vi "Calculate ANN.vi"(1 "1D ANN":i32[](array[numeric]), 2 "3D W":sgl[][][](array[numeric]) format="%.2f", 3 "Inputs":sgl[](array[numeric]) format="%.2f", 4 "Function":enum16{"Linear", "Sigmoid", "Tangent hyp."}(ring)) -> (7 "Neurons ouputs":sgl[][](array[numeric]) format="%.2f")   [LabVIEW 2010]
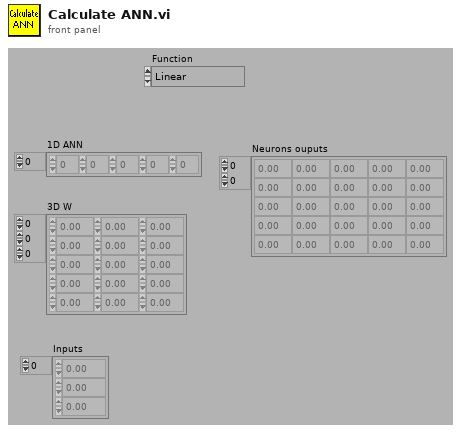
[diagram p1: front panel]
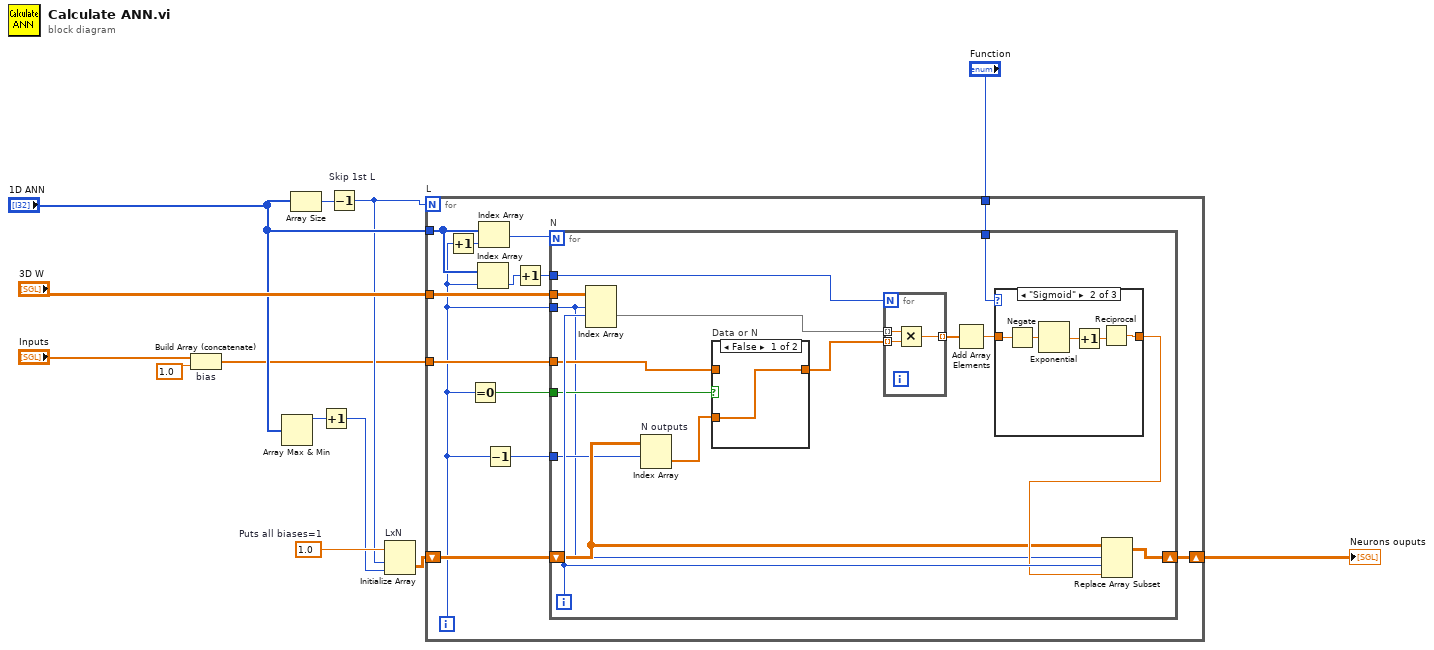
[diagram p0: block diagram]
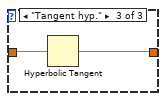
[diagram p3: hidden frame]
diagram:
  w7 = sgl 1.0  # Puts all biases=1
  n1 = Build Array (concatenate) "bias"("Inputs", sgl 1.0 ("Input Element")) -> (w1:sgl[])
  n2 = Array Max & Min(array="1D ANN") -> (max value=w5:i32)  [unwired: 3 out]
  n3 = Array Size(array="1D ANN") -> (size(s)=w8:i32)
  n4 = Increment(x=w5) -> (x+1=w3:i32)
  n5 = Decrement "Skip 1st L"(x=w8) -> (x-1=w6:i32)
  n6 = Initialize Array "LxN"(w7, w6, w3) -> (w4:sgl[][])
  n7 = for "L" {
    N: w6 -> [_]
    shift-right: [w26] -> w13
    shift-left: w4 -> [w16]
    tunnel: "1D ANN" -> [w20]
    tunnel: w1 -> [w22]
    tunnel: "Function" -> [w21]
    tunnel: "3D W" -> [w18]
    i -> [w14]
    n8 = Increment(x=w14) -> (x+1=w25:i32)
    n9 = Equal To 0?(x=w14) -> (x = 0?=w23:bool)
    n10 = Index Array(array=w20, index=w14) -> (element=w19:i32)
    n11 = Index Array(array=w20, index=w25) -> (element=w24:i32)
    n12 = Decrement(x=w14) -> (x-1=w15:i32)
    n13 = Increment(x=w19) -> (x+1=w17:i32)
    n14 = for "N" {
      N: w24 -> [_]
      shift-right: [w42] -> w26
      shift-left: w16 -> [w30]
      tunnel: w14 -> [w28]
      tunnel: w23 -> [w40]
      tunnel: w22 -> [w38]
      tunnel: w21 -> [w39]
      tunnel: w17 -> [w32]
      tunnel: w18 -> [w35]
      tunnel: w15 -> [w29]
      i -> [w41]
      n15 = Index Array(array=w35, index (dim 0)=w28, index (dim 1)=w41) -> (element=w34:sgl[])  [unwired: 1 in]
      n16 = Index Array "N outputs"(array=w30, index (row)=w29) -> (element=w33:sgl[])  [unwired: 1 in]
      n17 = case "Data or N" shown="False" w40 {
        tunnel: w33 -> [w54 _]
        tunnel: w38 -> [_ w55]
        tunnel: [w54 w55] -> w27
        frame False {
        }
        frame True {
        }
      }
      n18 = for {
        N: w32 -> [_]
        tunnel: [w45] -> w37 mode=indexing
        tunnel: w34 -> [w44] mode=indexing
        tunnel: w27 -> [w43] mode=indexing
        n19 = Multiply(x=w44, y=w43) -> (x*y=w45:sgl)
      }
      n20 = Add Array Elements(numeric array=w37) -> (sum=w36:sgl)
      n21 = case shown="\"Sigmoid\"" w39 {
        tunnel: w36 -> [w46 w48 w53]
        tunnel: [w46 w47 w52] -> w31
        frame "Linear", Default {
        }
        frame "Sigmoid" {
          n22 = Negate(x=w48) -> (-x=w51:sgl)
          n23 = Exponential(1:w51) -> (0:w50:sgl)
          n24 = Increment(x=w50) -> (x+1=w49:sgl)
          n25 = Reciprocal(x=w49) -> (1/x=w47:sgl)
        }
        frame "Tangent hyp." {
          n26 = Hyperbolic Tangent(1:w53) -> (0:w52:sgl)
        }
      }
      n27 = Replace Array Subset(array=w30, new element=w31, index (row)=w28, index (col)=w41) -> (w42:sgl[][])
    }
  }
  "Neurons ouputs" <- w13
